vi "Double FFT Mesurament (Max Bin detection - Control - Init Wave&Window - Snapshot - DoubleFFT) test.vi"() -> ()   [LabVIEW 2014]
uses:
  <vilib>/Platform/TimedLoop/XDataNode/timing_clust.ctl
  <vilib>/Platform/TimedLoop/XDataNode/nitl_modes.ctl
  <vilib>/Platform/TimedLoop/XDataNode/wakeup.ctl
  <vilib>/rvi/Analysis/measure/FFT/simModelSupport/niFPGA FFT Streaming Sim Properties.ctl
  <vilib>/rvi/Analysis/measure/FFT/simModelSupport/niFPGA FFT Sim Stream Group Properties.ctl
  <vilib>/rvi/Analysis/measure/FFT/simModelSupport/niFPGA FFT Sim Types.ctl
  <vilib>/rvi/Analysis/measure/FFT/simModelSupport/niFpgaFFTSimArithmeticProperties.ctl
  <vilib>/rvi/Analysis/measure/FFT/simModelSupport/niFpgaFFTSimDfxp.ctl
  <vilib>/fxp/LVFixedPointQuantizationPolicyTypeDef.ctl
  <vilib>/rvi/Analysis/measure/FFT/XNode/niFpgaFFTButterflyDelays.ctl
  <vilib>/rvi/Emulation/niFpgaSctlEmulationGetInTimedLoop.vi
  <vilib>/rvi/Emulation/niFpgaEmulationReportErrorSimple.vi
  <vilib>/rvi/Emulation/niFpgaGetClockAttributes.vi
  <vilib>/rvi/Emulation/niFpgaCriticalErrorInLSC.vi
  <vilib>/rvi/Emulation/niFpgaEmulationIsFPGAContextNoSignature.vi
  <vilib>/rvi/DataTransferAndStorage/Container/Common/niFpgaContainerGetUniqueNameForEmu.vi
  <vilib>/rvi/Memory/Memory_Emulation/niFpgaMemoryEmulationCacheClearOnFirstRun.vi
  <vilib>/rvi/Memory/Memory_Emulation/nirvimemoryEmulationManagerCache_MakeExclusive.vi
  <vilib>/rvi/Memory/Memory_Emulation/niFpgaMemoryEmulationValidateCache.vi
  <vilib>/rvi/Memory/Memory_Emulation/nirvimemoryEmulationManagerCache_InsertValue.vi
  <vilib>/Utility/error.llb/Clear Errors.vi
  <vilib>/rvi/Memory/Memory_Emulation/nirvimemoryEmulationManagerCache_ReleaseExclusive.vi
  <vilib>/rvi/Memory/Memory_Emulation/nirvimemoryEmulationManagerCache_GetValue.vi
  <vilib>/rvi/Memory/Memory_Emulation/nirvimemoryEmulationManagerCache_SetValue.vi
  <vilib>/rvi/Emulation/niFpgaProcessEmulError.vi
  <vilib>/rvi/errors/niFpgaSetErrorForExecOnDevCompSimple.vi
  <vilib>/rvi/eio/common/nirviEmuReportErrorAndStop.vi
  <vilib>/rvi/FIFO/Fifo_Resource/nirvififoEmulationSetSize.vi
  <vilib>/rvi/FIFO/Fifo_Resource/nirviFifoEmulationQueueMgr.vi
  <instcachedir>/0/nirviFifoEmulationQueueMgr_E5CAEC123FF24DC58D834DCA3CDAA9B5.lvgen/nirviFifoEmulationQueueMgr_E5CAEC123FF24DC58D834DCA3CDAA9B5_012.vi
  <vilib>/rvi/FIFO/Fifo_Resource/nirvififoEmulationCreateLock.vi
  <vilib>/rvi/FIFO/Fifo_Resource/nirvififoEmulationObtainLock.vi
  <vilib>/rvi/FIFO/Fifo_Resource/nirvififoEmulationReleaseLock.vi
  <vilib>/rvi/occurrence/nirviWaitOnOccurrenceBase.vi
  <vilib>/rvi/errors/nirviReportUnexpectedCaseInternalError.vi
  <vilib>/rvi/errors/nirviReportUnexpectedCaseInternalError (U32).vi
  <instcachedir>/0/nirviFifoEmulationQueueMgr_E5CAEC123FF24DC58D834DCA3CDAA9B5.lvgen/nirviFifoEmulationQueueMgr_E5CAEC123FF24DC58D834DCA3CDAA9B5_010.vi
  <vilib>/rvi/FIFO/Fifo_Resource/nirvififoEmulationDetermineInputValidOut.vi
  <vilib>/rvi/Memory/Memory_Emulation/nirvimemoryFastEmulation.vi
  <vilib>/rvi/Memory/Memory_Emulation/nirvimemoryEmulation.vi
  <vilib>/rvi/Analysis/measure/FFT/simModelSupport/niFpgaFFTSimModelStreamingCore.vi
  <vilib>/rvi/interface/RandomDataEmulation/niFpgaRandomDataHandleErrors.vi
  <vilib>/rvi/eio/common/nirviEmuTemplateMethod_errors.vi
  <vilib>/Platform/TimedLoop/XDataNode/XDataNode.xnode
  <vilib>/rvi/DataTransferAndStorage/Container/XNode/niFpgaContainer.xnode
  <vilib>/rvi/DataTransferAndStorage/Register/Emulation/niFpgaRegisterEmulation.vi
  <vilib>/rvi/FIFO/Fifo_Resource/nirvififoEmulationRead.vi
  <vilib>/rvi/FIFO/Fifo_Resource/nirvififoEmulationWrite.vi
  <vilib>/rvi/FIFO/Fifo_Resource/nirvififoEmulationGetNumberOfElementsToWrite.vi
  <vilib>/rvi/Analysis/measure/FFT/XNode/niFpgaFFT.xnode
  <vilib>/rvi/interface/RandomDataEmulation/nirviRandomDataFpgaReadWriteTemplate.vi
  <vilib>/eio/EIOMethodNode/EIOMethodNode.xnode
  <vilib>/Platform/TimedLoop/XDataNode/XDNodeRunTimeDep.lvlib
panel:
  in  "snapshot":bool
  in  "first bin":i32=4
  in  "last bin":i32=251
  in  "lower limit 2":u32=682
  in  "lower limit 1":u32=57
  in  "upper limit 2":u32=1193
  in  "upper limit 1":u32=568
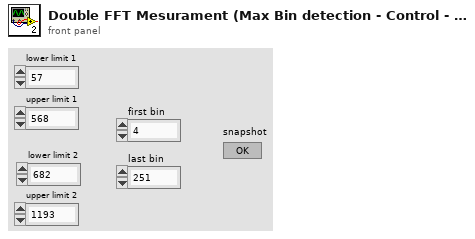
[diagram p1: front panel]
types:
  T1 = typedef "XDNodeRunTimeDep.lvlib/timing_clust.ctl" = cluster{"Expected End [f-1]":u64, "Actual End [f-1]":u64, "Finished Late? [f-1]":bool, "Expected End [i-1]":u64, "Actual End [i-1]":u64, "Finished Late? [i-1]":bool, "Expected Start [i]":u64, "Actual Start [i]":u64, "Expected Start [f]":u64, "Actual Start [f]":u64, "Source Name":string, "Structure Name":string, "Period":i64, "Deadline":i64, "Offset":i64, "Start":i64, "Priority":i32, "Timeout":i32, "Mode":T2, "Wakeup Reason":T3, "Error":errorcluster, "Source Type":string, "Secondary Source Type":string, "Global End Time":u64, "Global Start Time":u64, "Frame Duration":u64, "Iteration Duration":u64, "Assigned CPU":i32, "I/O Scan Engine Mode":u32}
  T2 = typedef "XDNodeRunTimeDep.lvlib/nitl_modes.ctl" = enum32{"No Change", "Process missed periods, maintain original phase", "Discard missed periods, maintain original phase", "Process missed periods, ignore original phase", "Discard missed periods, ignore original phase"}
  T3 = typedef "XDNodeRunTimeDep.lvlib/wakeup.ctl" = enum32{"Normal", "Aborted", "Asynchronous wakeup", "Timing source error", "Timed loop error", "Timeout"}
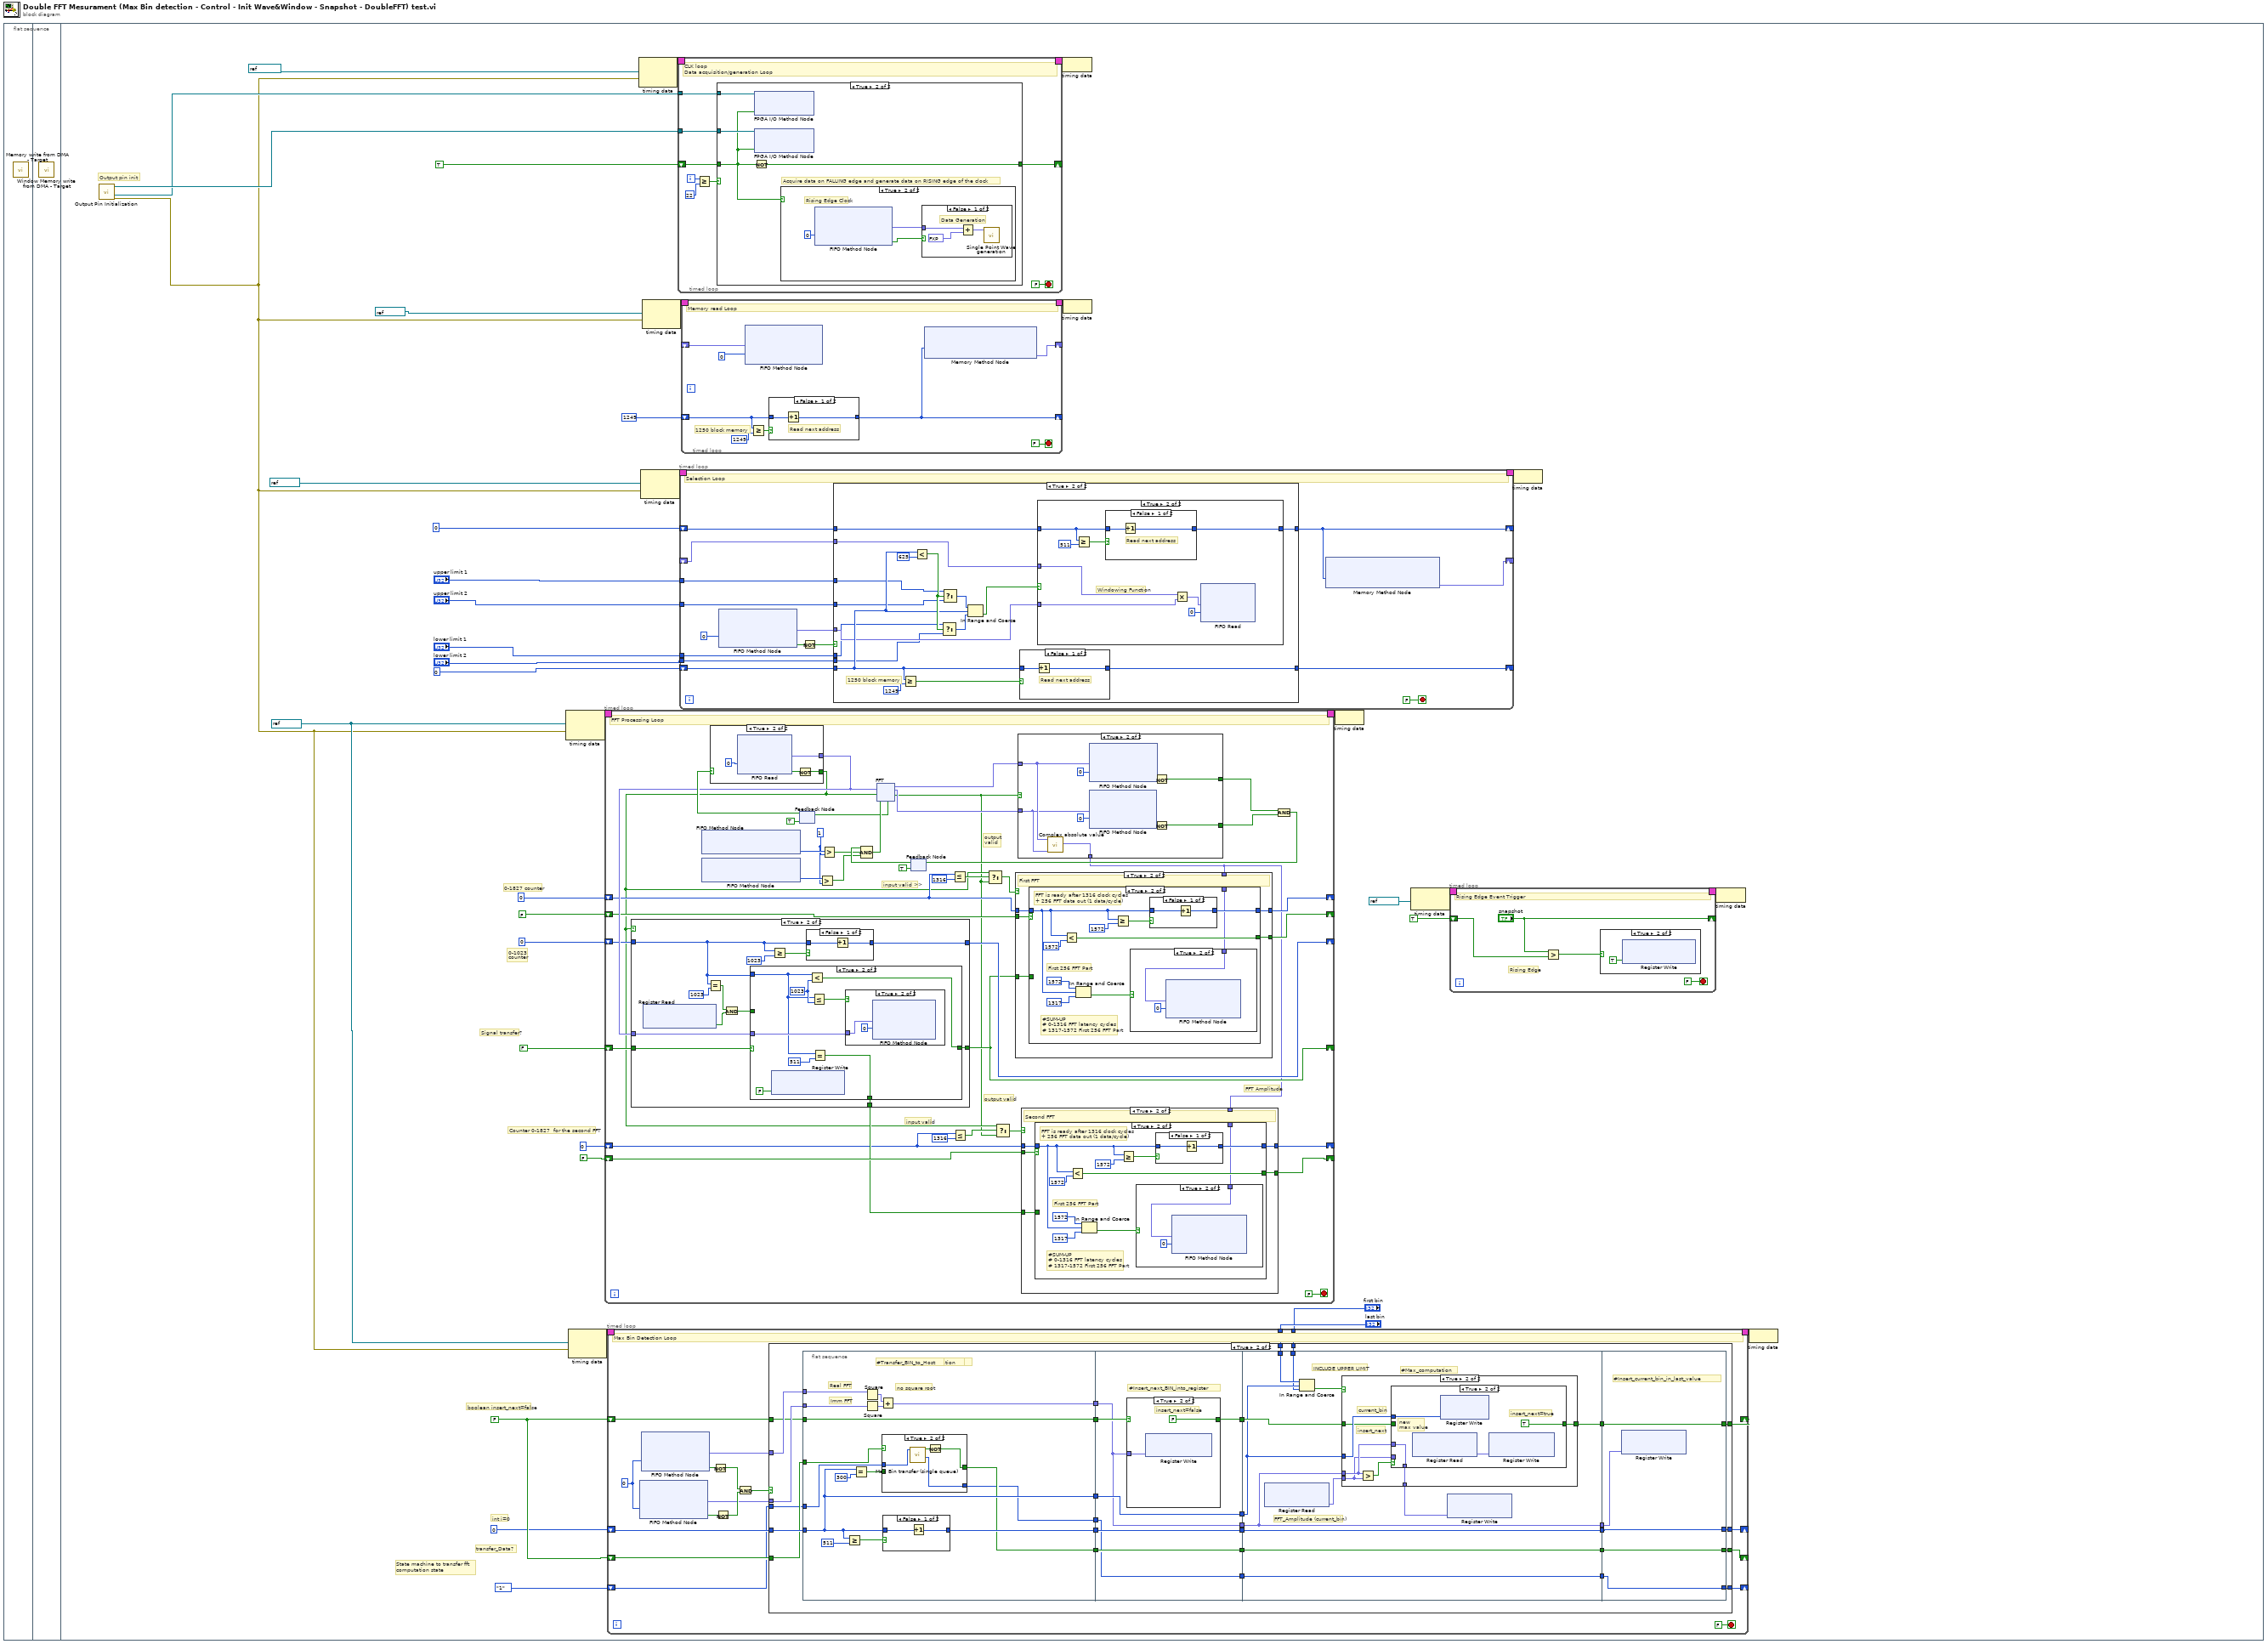
[diagram p0: block diagram]
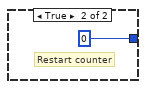
[diagram p5: hidden frame]
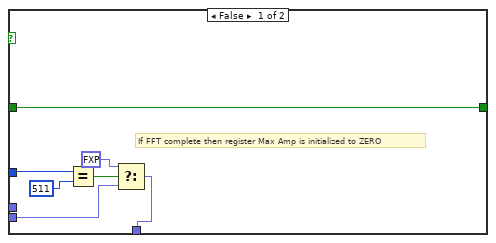
[diagram p7: hidden frame]
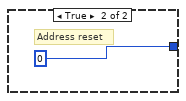
[diagram p11: hidden frame]
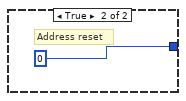
[diagram p12: hidden frame]
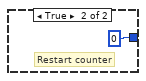
[diagram p16: hidden frame]
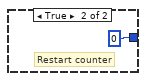
[diagram p20: hidden frame]
diagram:
  n1 = flat-sequence {
    frame #0 {
      n2 = call "Memory write from DMA - Target.vi"() -> ()  [unwired: 12 in]
    }
    frame #1 {
      n3 = call "Window Memory write from DMA - Target.vi"() -> ()  [unwired: 12 in]
    }
    frame #2 {
      w13 = FALSE
      w22 = refnum<k21> "50MHz" ("Source Name")
      # "Counter 0-1827  for the second FFT"
      # "0-1827 counter"
      # "0-1023\ncounter"
      # "Signal transfer?"
      # "State machine to transfer fft\ncomputation state"
      # "transfer_Data?"
      # "int i=0"
      # "boolean insert_next=false"
      # "Output pin init"
      n4 = call "Output Pin Initialization.vi"() -> ("error out"=w21:errorcluster, "I/O Out Clock DAC (pin16)"=w25:refnum<k21>, "I/O Out Clock ADC (pin17)"=w26:refnum<k21>)  [unwired: 8 in]
      n5 = node-c288(w22, w21) -> (w36:T1)
      n6 = node-c288(w22, w21) -> (w32:T1)
      n7 = timed-loop {
        timing: w36 -> [_]
        timing-out: [_] -> w35
        shift-right: [w257] -> _
        shift-left: FALSE -> [w260]
        shift-right: [w261] -> _
        shift-left: i16 0 -> [w258]
        shift-right: [w256] -> _
        shift-left: FALSE -> [w255]
        shift-right: [w254] -> _
        shift-left: i16 0 -> [w252]
        shift-right: [w249] -> _
        shift-left: i16 0 -> [w242]
        shift-right: [w246] -> _
        shift-left: FALSE -> [w247]
        stop <- FALSE stop-if-true
        w264 = u32 1 ("y")
        # "output valid"
        # "input valid"
        # "FFT Amplitude"
        # "output\nvalid"
        # "input valid >>"
        # "FFT Processing Loop"
        n8 = xnode ("FIFO Method Node")() -> ("Number of Elements to Write"=w266:u32)  [unwired: 1 in, 1 out]
        n9 = xnode ("FIFO Method Node")() -> ("Number of Elements to Write"=w265:u32)  [unwired: 1 in, 1 out]
        n10 = feedback #1(TRUE ("ready for input")) -> (w278:bool)
        n11 = case shown="True" w278 {
          tunnel: [FALSE w400] -> w241
          tunnel: [fxp<+/-,12,12> 0.0 ("Element") w397] -> w259
          frame False {
            # "RMS is not ready for new input"
          }
          frame True {
            n12 = xnode ("FIFO Read")("Timeout"=0) -> ("Element"=w397:fxp<+/-,12,12>, "Timed Out?"=w399:bool)  [unwired: 1 in, 1 out]
            n13 = Not(x=w399) -> (.not. x?=w400:bool)
          }
        }
        n14 = case shown="True" w241 {
          tunnel: w258 -> [w331 w337]
          tunnel: [w331 w341] -> w261
          tunnel: w260 -> [w330 w335]
          tunnel: [w330 w336] -> w257
          tunnel: w259 -> [_ w334]
          tunnel: [FALSE w332] -> w245
          frame False {
          }
          frame True {
            n15 = xnode ("Register Read")() -> ("Data"=w333:bool)  [unwired: 1 in, 1 out]
            n16 = Equal?(x=w337, y=i16 1023) -> (x = y?=w340:bool)
            n17 = And(x=w340, y=w333) -> (x .and. y?=w338:bool)
            n18 = case shown="True" w335 {
              tunnel: w338 -> [w345 _]
              tunnel: w337 -> [_ w348]
              tunnel: [w345 w353] -> w336
              tunnel: w334 -> [_ w351]
              tunnel: [FALSE w346] -> w332
              frame False {
              }
              frame True {
                w350 = i16 1023 ("y")
                n19 = xnode ("Register Write")("Data"=FALSE) -> ()  [unwired: 1 in, 1 out]
                n20 = Less?(x=w348, y=w350) -> (x < y?=w353:bool)
                n21 = Less Or Equal?(x=w348, y=w350) -> (x <= y?=w352:bool)
                n22 = Equal?(x=w348, y=i16 511) -> (x = y?=w346:bool)
                n23 = case shown="True" w352 {
                  tunnel: w351 -> [_ w354]
                  frame False {
                  }
                  frame True {
                    n24 = xnode ("FIFO Method Node")("Element"=w354, "Timeout"=0) -> ()  [unwired: 1 in, 2 out]
                  }
                }
              }
            }
            n25 = Greater Or Equal?(x=w337, y=i16 1023) -> (x >= y?=w342:bool)
            n26 = case shown="False" w342 {
              tunnel: w337 -> [w357 _]
              tunnel: [w356 i16 0] -> w341
              frame False {
                n27 = Increment(x=w357) -> (x+1=w356:i16)
              }
              frame True {
                # "Restart counter"
              }
            }
          }
        }
        n28 = Greater?(x=w265, y=w264) -> (0:w262:bool)
        n29 = Greater?(x=w266, y=w264) -> (0:w263:bool)
        n30 = feedback #2(TRUE) -> (w274:bool)
        n31 = Compound Arithmetic op=AND(w274, w263, w262) -> (w273:bool)
        n32 = xnode "FFT"("real data in"=w259, "input valid"=w241, "ready for output"=w273) -> ("ready for input"=w272:bool, "real data out"=w271:fxp<+/-,22,22>, "imaginary data out"=w270:fxp<+/-,22,22>, "output valid"=w239:bool)  [unwired: 2 in, 1 out]
        n33 = feedback-in #1(w272) -> ()
        n34 = Less Or Equal?(x=w252, y=i16 1316) -> (x <= y?=w253:bool)
        n35 = Less Or Equal?(x=w242, y=i16 1316) -> (x <= y?=w243:bool)
        n36 = Select(t=w241, s=w253, f=w239) -> (s? t:f=w250:bool)
        n37 = Select(t=w241, s=w243, f=w239) -> (s? t:f=w240:bool)
        n38 = case shown="True" w239 {
          tunnel: w271 -> [_ w388]
          tunnel: w270 -> [_ w387]
          tunnel: [w385 w394] -> w269
          tunnel: [w385 w393] -> w268
          tunnel: [_ w386] -> w248
          frame False {
            w385 = TRUE
          }
          frame True {
            n39 = call "Complex absolute value.vi"("Im"=w387, "Re"=w388) -> ("Square Absolute Value"=w386:fxp<+,44,44>)  [unwired: 9 in]
            n40 = xnode ("FIFO Method Node")("Element"=w388, "Timeout"=0) -> ("Timed Out?"=w389:bool)  [unwired: 1 in, 1 out]
            n41 = xnode ("FIFO Method Node")("Element"=w387, "Timeout"=0) -> ("Timed Out?"=w390:bool)  [unwired: 1 in, 1 out]
            n42 = Not(x=w389) -> (.not. x?=w394:bool)
            n43 = Not(x=w390) -> (.not. x?=w393:bool)
          }
        }
        n44 = case shown="True" w250 {
          tunnel: w257 -> [_ w311]
          tunnel: [w304 w310] -> w256
          tunnel: w255 -> [w304 w309]
          tunnel: w252 -> [w305 w308]
          tunnel: [w305 w307] -> w254
          tunnel: w248 -> [_ w306]
          frame False {
          }
          frame True {
            # "First FFT"
            n45 = case shown="True" w309 {
              tunnel: w311 -> [w313 _]
              tunnel: [w313 w323] -> w310
              tunnel: w308 -> [w312 w316]
              tunnel: [w312 w319] -> w307
              tunnel: w306 -> [_ w314]
              frame False {
              }
              frame True {
                # "First 256 FFT Part"
                # "#SUM-UP\n# 0-1316 FFT latency cycles\n# 1317-1572 First 256 FFT Part"
                # "FFT is ready after 1316 clock cycles\n+ 256 FFT data out (1 data/cycle)"
                n46 = Less?(x=w316, y=i16 1572) -> (x < y?=w323:bool)
                n47 = In Range and Coerce(upper limit=i16 1572, x=w316, lower limit=i16 1317 ("y")) -> (In Range?=w315:bool)  [unwired: 1 out]
                n48 = Greater Or Equal?(x=w316, y=i16 1572) -> (x >= y?=w320:bool)
                n49 = case shown="True" w315 {
                  tunnel: w314 -> [_ w325]
                  frame False {
                  }
                  frame True {
                    n50 = xnode ("FIFO Method Node")("Element"=w325, "Timeout"=0) -> ()  [unwired: 1 in, 2 out]
                  }
                }
                n51 = case shown="False" w320 {
                  tunnel: w316 -> [w327 _]
                  tunnel: [w326 i16 0] -> w319
                  frame False {
                    n52 = Increment(x=w327) -> (x+1=w326:i16)
                  }
                  frame True {
                    # "Restart counter"
                  }
                }
              }
            }
          }
        }
        n53 = case shown="True" w240 {
          tunnel: w245 -> [_ w286]
          tunnel: [w279 w285] -> w246
          tunnel: w247 -> [w279 w284]
          tunnel: w242 -> [w280 w283]
          tunnel: [w280 w282] -> w249
          tunnel: w248 -> [_ w281]
          frame False {
          }
          frame True {
            # "Second FFT"
            n54 = case shown="True" w284 {
              tunnel: w286 -> [w288 _]
              tunnel: [w288 w298] -> w285
              tunnel: w283 -> [w287 w291]
              tunnel: [w287 w294] -> w282
              tunnel: w281 -> [_ w289]
              frame False {
              }
              frame True {
                # "First 256 FFT Part"
                # "#SUM-UP\n# 0-1316 FFT latency cycles\n# 1317-1572 First 256 FFT Part"
                # "FFT is ready after 1316 clock cycles\n+ 256 FFT data out (1 data/cycle)"
                n55 = Less?(x=w291, y=i16 1572) -> (x < y?=w298:bool)
                n56 = In Range and Coerce(upper limit=i16 1572, x=w291, lower limit=i16 1317 ("y")) -> (In Range?=w290:bool)  [unwired: 1 out]
                n57 = Greater Or Equal?(x=w291, y=i16 1572) -> (x >= y?=w295:bool)
                n58 = case shown="True" w290 {
                  tunnel: w289 -> [_ w300]
                  frame False {
                  }
                  frame True {
                    n59 = xnode ("FIFO Method Node")("Element"=w300, "Timeout"=0) -> ()  [unwired: 1 in, 2 out]
                  }
                }
                n60 = case shown="False" w295 {
                  tunnel: w291 -> [w302 _]
                  tunnel: [w301 i16 0] -> w294
                  frame False {
                    n61 = Increment(x=w302) -> (x+1=w301:i16)
                  }
                  frame True {
                    # "Restart counter"
                  }
                }
              }
            }
          }
        }
        n62 = Compound Arithmetic op=AND(w269, w268) -> (w267:bool)
        n63 = feedback-in #2(w267) -> ()
      }
      n64 = timed-loop {
        shift-right: [w62] -> _
        shift-left: 0 ("Timeout") -> [w63]
        shift-right: [w60] -> _
        shift-left: w13 -> [w61]
        timing: w32 -> [_]
        timing-out: [_] -> w31
        tunnel: "last bin" -> [w58]
        tunnel: "first bin" -> [w57]
        shift-right: [w54] -> _
        shift-left: w13 -> [w55]
        shift-right: [w52] -> _
        shift-left: enum16{"1", "2", "3", "4"}."1" ("Enum") -> [w53]
        stop <- FALSE stop-if-true
        w56 = 0 ("Timeout")
        # "Max Bin Detection Loop"
        n65 = xnode ("FIFO Method Node")("Timeout"=w56) -> ("Element"=w64:fxp<+/-,22,22>, "Timed Out?"=w69:bool)  [unwired: 1 in, 1 out]
        n66 = xnode ("FIFO Method Node")("Timeout"=w56) -> ("Element"=w65:fxp<+/-,22,22>, "Timed Out?"=w70:bool)  [unwired: 1 in, 1 out]
        n67 = Not(x=w70) -> (.not. x?=w68:bool)
        n68 = Not(x=w69) -> (.not. x?=w67:bool)
        n69 = And(x=w68, y=w67) -> (x .and. y?=w66:bool)
        n70 = case shown="True" w66 {
          tunnel: w65 -> [_ w103]
          tunnel: w64 -> [_ w102]
          tunnel: w63 -> [w74 w100]
          tunnel: [w74 w87] -> w62
          tunnel: w61 -> [w73 w94]
          tunnel: [w73 w89] -> w60
          tunnel: w58 -> [_ w86]
          tunnel: w57 -> [_ w85]
          tunnel: w55 -> [w72 w84]
          tunnel: [w72 w83] -> w54
          tunnel: w53 -> [w71 w79]
          tunnel: [w71 w75] -> w52
          frame False {
            # "Data are NOT ready in Target Real FFT and Target Imm FFT FIFOs"
          }
          frame True {
            n71 = flat-sequence {
              tunnel: w103 -> [w116]
              tunnel: w102 -> [w117]
              tunnel: [w110] -> w101
              tunnel: w100 -> [w109]
              tunnel: [w115] -> w99
              tunnel: [w109] -> w96
              tunnel: [w112] -> w95
              tunnel: w94 -> [w112]
              tunnel: w84 -> [w108]
              tunnel: [w106] -> w82
              tunnel: w79 -> [w105]
              tunnel: [w104] -> w76
              tunnel: w101 -> [w132]
              tunnel: w99 -> [w135]
              tunnel: [w135] -> w98
              tunnel: w96 -> [w133]
              tunnel: w95 -> [w134]
              tunnel: [w133] -> w93
              tunnel: [w132] -> w92
              tunnel: [w131] -> w91
              tunnel: w82 -> [w130]
              tunnel: [w130] -> w81
              tunnel: [w129] -> w77
              tunnel: w76 -> [w129]
              tunnel: w98 -> [w150]
              tunnel: [w150] -> w97
              tunnel: w93 -> [w145]
              tunnel: w92 -> [w147]
              tunnel: w91 -> [w148]
              tunnel: [w147] -> w90
              tunnel: [w146] -> w88
              tunnel: w86 -> [w142]
              tunnel: w85 -> [w141]
              tunnel: w81 -> [w140]
              tunnel: [w140] -> w80
              tunnel: [w139] -> w78
              tunnel: w77 -> [w139]
              tunnel: w97 -> [w173]
              tunnel: w90 -> [w175]
              tunnel: w88 -> [w174]
              tunnel: [w174] -> w89
              tunnel: [w173] -> w87
              tunnel: [w172] -> w83
              tunnel: w80 -> [w172]
              tunnel: w78 -> [w171]
              tunnel: [w171] -> w75
              frame #0 {
                # "no square root"
                # "#Transfer_BIN_to_Host"
                # "#Iteration_Counter_Computation"
                # "#FFT_Amplitude_Computation"
                # "Imm FFT"
                # "Real FFT"
                n72 = Greater Or Equal?(x=w109, y=511) -> (x >= y?=w113:bool)
                n73 = Equal?(x=w109, y=300) -> (x = y?=w107:bool)
                n74 = Square(x=w116) -> (x^2=w119:fxp<+,43,43>)
                n75 = Square(x=w117) -> (x^2=w118:fxp<+,43,43>)
                n76 = Add(x=w119, y=w118) -> (x+y=w110:fxp<+,44,44>)
                n77 = case shown="True" w108 {
                  tunnel: w107 -> [w121 _]
                  tunnel: [w121 w124] -> w106
                  tunnel: w105 -> [w120 w123]
                  tunnel: [w120 w122] -> w104
                  frame False {
                    # "FFT Comp is NOT finished"
                  }
                  frame True {
                    n78 = call "Max Bin transfer (single queue).vi"("Enum"=w123) -> ("Next state"=w122:enum16{"1", "2", "3", "4"}, "END?"=w125:bool)  [unwired: 9 in]
                    n79 = Not(x=w125) -> (.not. x?=w124:bool)
                  }
                }
                n80 = case shown="False" w113 {
                  tunnel: w109 -> [w126 _]
                  tunnel: [w127 0 ("Timeout")] -> w115
                  frame False {
                    n81 = Increment(x=w126) -> (x+1=w127:i32)
                  }
                  frame True {
                    # "Restart counter"
                  }
                }
              }
              frame #1 {
                # "#Insert_next_BIN_into_register"
                n82 = case shown="True" w134 {
                  selector: w134 -> [w136 _]
                  tunnel: [w136 FALSE] -> w131
                  tunnel: w132 -> [_ w137]
                  frame False {
                  }
                  frame True {
                    # "insert_next=false"
                    n83 = xnode ("Register Write")("Data"=w137) -> ()  [unwired: 1 in, 1 out]
                  }
                }
              }
              frame #2 {
                # "INCLUDE UPPER LIMIT"
                # "FFT_Amplitude (current_bin)"
                # "#Max_computation"
                n84 = xnode ("Register Read")() -> ("Data"=w144:fxp<+,44,44>)  [unwired: 1 in, 1 out]
                n85 = In Range and Coerce(upper limit=w142, x=w145, lower limit=w141) -> (In Range?=w149:bool)  [unwired: 1 out]
                n86 = case shown="True" w149 {
                  tunnel: w147 -> [_ w163]
                  tunnel: w145 -> [w155 w162]
                  tunnel: w148 -> [w157 w161]
                  tunnel: [w157 w160] -> w146
                  tunnel: w144 -> [w153 w158]
                  tunnel: [w151 w159] -> w143
                  frame False {
                    # "If FFT complete then register Max Amp is initialized to ZERO"
                    n87 = Equal?(x=w155, y=511) -> (x = y?=w156:bool)
                    n88 = Select(t=fxp<+,44,44> 0.0, s=w156, f=w153) -> (s? t:f=w151:fxp<+,44,44>)
                  }
                  frame True {
                    # "insert_next"
                    # "current_bin"
                    n89 = Greater?(x=w163, y=w158) -> (0:w164:bool)
                    n90 = case shown="True" w164 {
                      tunnel: w163 -> [_ w167]
                      tunnel: w162 -> [_ w170]
                      tunnel: w161 -> [w166 _]
                      tunnel: [w166 TRUE] -> w160
                      tunnel: [w165 w167] -> w159
                      tunnel: w158 -> [w165 _]
                      frame False {
                        # "Old value is re-written"
                      }
                      frame True {
                        # "new\nmax value"
                        # "insert_next=true"
                        n91 = xnode ("Register Read")() -> ("Data"=w168:fxp<+,44,44>)  [unwired: 1 in, 1 out]
                        n92 = xnode ("Register Write")("Data"=w170) -> ()  [unwired: 1 in, 1 out]
                        n93 = xnode ("Register Write")("Data"=w168) -> ()  [unwired: 1 in, 1 out]
                      }
                    }
                  }
                }
                n94 = xnode ("Register Write")("Data"=w143) -> ()  [unwired: 1 in, 1 out]
              }
              frame #3 {
                # "#Insert_current_bin_in_last_value"
                n95 = xnode ("Register Write")("Data"=w175) -> ()  [unwired: 1 in, 1 out]
              }
            }
          }
        }
      }
      n96 = node-c288(refnum<k21> "100MHz" ("Source Name"), w21) -> (w40:T1)
      n97 = node-c288(refnum<k21> "50MHz" ("Source Name"), w21) -> (w34:T1)
      n98 = node-c288(refnum<k21> "50MHz" ("Source Name"), w21) -> (w38:T1)
      n99 = timed-loop {
        timing: w40 -> [_]
        timing-out: [_] -> w39
        shift-right: [w431] -> _
        shift-left: TRUE -> [w429]
        tunnel: w25 -> [w433]
        tunnel: w26 -> [w430]
        i -> [w428]
        stop <- FALSE stop-if-true
        # "CLK loop\nData acquisition/generation Loop"
        n100 = Greater Or Equal?(x=w428, y=22) -> (x >= y?=w426:bool)
        n101 = case shown="True" w426 {
          tunnel: w433 -> [_ w438]
          tunnel: [w434 w437] -> w431
          tunnel: w430 -> [_ w436]
          tunnel: w429 -> [w434 w435]
          frame False {
          }
          frame True {
            # "Acquire data on FALLING edge and generate data on RISING edge of the clock"
            n102 = Not(x=w435) -> (.not. x?=w437:bool)
            n103 = xnode "FPGA I/O Method Node"("FPGA I/O In"=w438, "Data"=w435) -> ()  [unwired: 1 out]
            n104 = xnode "FPGA I/O Method Node"("FPGA I/O In"=w436, "Data"=w435) -> ()  [unwired: 1 out]
            n105 = case shown="True" w435 {
              frame False {
                # "Falling Edge Clock"
                n106 = call "Single Acquisition.vi"() -> ("Out"=w440:fxp<+/-,12,12>)  [unwired: 10 in, 1 out]
                n107 = xnode ("FIFO Method Node")("Element"=w440, "Timeout"=0) -> ()  [unwired: 1 in, 2 out]
              }
              frame True {
                # "Rising Edge Clock"
                n108 = xnode ("FIFO Method Node")("Timeout"=0) -> ("Element"=w441:fxp<+/-,12,12>, "Timed Out?"=w442:bool)  [unwired: 1 in, 1 out]
                n109 = case shown="False" w442 {
                  tunnel: w441 -> [w446 _]
                  frame False {
                    # "Data Generation"
                    n110 = Add(x=w446, y=fxp<+,12,12> 2048.0) -> (x+y=w444:fxp<+/-,14,14>)
                    n111 = call "Single Point Wave generation.vi"("Data To Write"=w444) -> ()  [unwired: 10 in, 1 out]
                  }
                  frame True {
                    # "FPGA memory slow"
                  }
                }
              }
            }
          }
        }
      }
      n112 = timed-loop {
        timing: w34 -> [_]
        timing-out: [_] -> w33
        shift-right: [w196] -> _
        shift-left: u32 0 -> [w195]
        tunnel: "upper limit 1" -> [w190]
        tunnel: "upper limit 2" -> [w189]
        tunnel: "lower limit 1" -> [w188]
        tunnel: "lower limit 2" -> [w187]
        shift-right: [w183] -> _
        shift-left: u32 0 -> [w186]
        shift-right: [w184] -> _
        shift-left: _ -> [w185]
        stop <- FALSE stop-if-true
        # "Selection Loop"
        n113 = xnode ("FIFO Method Node")("Timeout"=0) -> ("Element"=w192:fxp<+/-,12,12>, "Timed Out?"=w193:bool)  [unwired: 1 in, 1 out]
        n114 = Not(x=w193) -> (.not. x?=w194:bool)
        n115 = case shown="True" w194 {
          tunnel: [w199 w214] -> w196
          tunnel: w195 -> [w199 w209]
          tunnel: w192 -> [_ w207]
          tunnel: w190 -> [_ w206]
          tunnel: w189 -> [_ w205]
          tunnel: w188 -> [_ w204]
          tunnel: w187 -> [_ w203]
          tunnel: w186 -> [w198 w200]
          tunnel: [w198 w202] -> w183
          tunnel: w185 -> [_ w201]
          frame False {
          }
          frame True {
            # "1250 block memory"
            n116 = Greater Or Equal?(x=w209, y=u32 1249) -> (x >= y?=w215:bool)
            n117 = Less?(x=w209, y=u32 625) -> (x < y?=w210:bool)
            n118 = Select(t=w204, s=w210, f=w203) -> (s? t:f=w212:u32)
            n119 = Select(t=w206, s=w210, f=w205) -> (s? t:f=w213:u32)
            n120 = In Range and Coerce(upper limit=w213, x=w209, lower limit=w212) -> (In Range?=w208:bool)  [unwired: 1 out]
            n121 = case shown="False" w215 {
              tunnel: w209 -> [w230 _]
              tunnel: [w229 u32 0] -> w214
              frame False {
                # "Read next address"
                n122 = Increment(x=w230) -> (x+1=w229:u32)
              }
              frame True {
                # "Address reset"
              }
            }
            n123 = case shown="True" w208 {
              tunnel: w207 -> [_ w218]
              tunnel: w200 -> [w217 w223]
              tunnel: [w217 w225] -> w202
              tunnel: w201 -> [_ w221]
              frame False {
              }
              frame True {
                # "Windowing Function"
                n124 = Greater Or Equal?(x=w223, y=u32 511) -> (x >= y?=w224:bool)
                n125 = case shown="False" w224 {
                  tunnel: w223 -> [w227 _]
                  tunnel: [w226 u32 0] -> w225
                  frame False {
                    # "Read next address"
                    n126 = Increment(x=w227) -> (x+1=w226:u32)
                  }
                  frame True {
                    # "Address reset"
                  }
                }
                n127 = Multiply(x=w221, y=w218) -> (x*y=w219:fxp<+/-,12,12>)
                n128 = xnode ("FIFO Read")("Element"=w219, "Timeout"=0) -> ()  [unwired: 1 in, 2 out]
              }
            }
          }
        }
        n129 = xnode ("Memory Method Node")("Address"=w183) -> ("Data"=w184:fxp<+,8,1>)  [unwired: 1 in, 1 out]
      }
      n130 = timed-loop {
        timing: w38 -> [_]
        timing-out: [_] -> w37
        shift-right: [w408] -> _
        shift-left: u32 1249 -> [w412]
        shift-right: [w410] -> _
        shift-left: _ -> [w409]
        stop <- FALSE stop-if-true
        # "1250 block memory"
        # "Memory read Loop"
        n131 = xnode ("FIFO Method Node")("Element"=w409, "Timeout"=0) -> ()  [unwired: 1 in, 2 out]
        n132 = Greater Or Equal?(x=w412, y=u32 1249) -> (x >= y?=w414:bool)
        n133 = case shown="False" w414 {
          tunnel: w412 -> [w417 _]
          tunnel: [w416 u32 0] -> w408
          frame False {
            # "Read next address"
            n134 = Increment(x=w417) -> (x+1=w416:u32)
          }
          frame True {
            # "Address reset"
          }
        }
        n135 = xnode ("Memory Method Node")("Address"=w408) -> ("Data"=w410:fxp<+/-,12,12>)  [unwired: 1 in, 1 out]
      }
      n136 = node-c288(w39) -> ()
      n137 = node-c288(w37) -> ()
      n138 = node-c288(w35) -> ()
      n139 = node-c288(refnum<k21> "50MHz" ("Source Name")) -> (w6:T1)
      n140 = timed-loop {
        timing: w6 -> [_]
        timing-out: [_] -> w5
        shift-right: ["snapshot"] -> _
        shift-left: TRUE ("snapshot") -> [w43]
        stop <- FALSE stop-if-true
        # "Rising Edge"
        # "Rising Edge Event Trigger"
        n141 = Greater?(x="snapshot", y=w43) -> (0:w41:bool)
        n142 = case shown="True" w41 {
          frame False {
          }
          frame True {
            n143 = xnode ("Register Write")("Data"=TRUE) -> ()  [unwired: 1 in, 1 out]
          }
        }
      }
      n144 = node-c288(w33) -> ()
      n145 = node-c288(w5) -> ()
      n146 = node-c288(w31) -> ()
    }
  }
